vi "Send SMS 2012.vi"(4 "Body":string, 5 "Carrier":enum16{"T-Mobile", "AT&T", "Verizon", "Sprint"}(ring), 6 "Subject":string, 7 "phone number":string, 8 "Error In":errorcluster, 9 "smtp server":string="smtp.gmail.com", 10 "password":string, 11 "email username":string) -> (0 "Error Out":errorcluster)   [LabVIEW 2012]
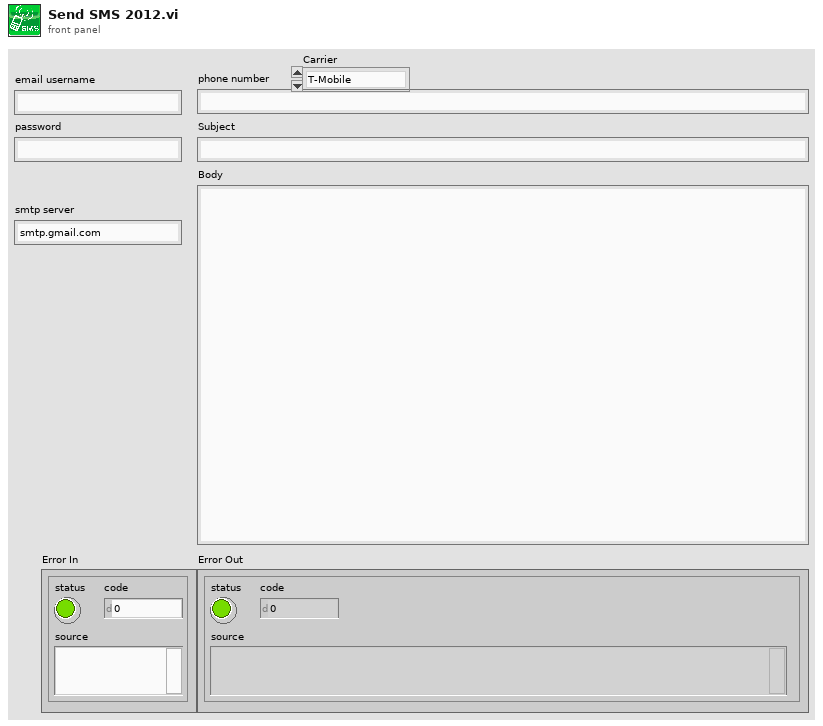
[diagram p1: front panel]
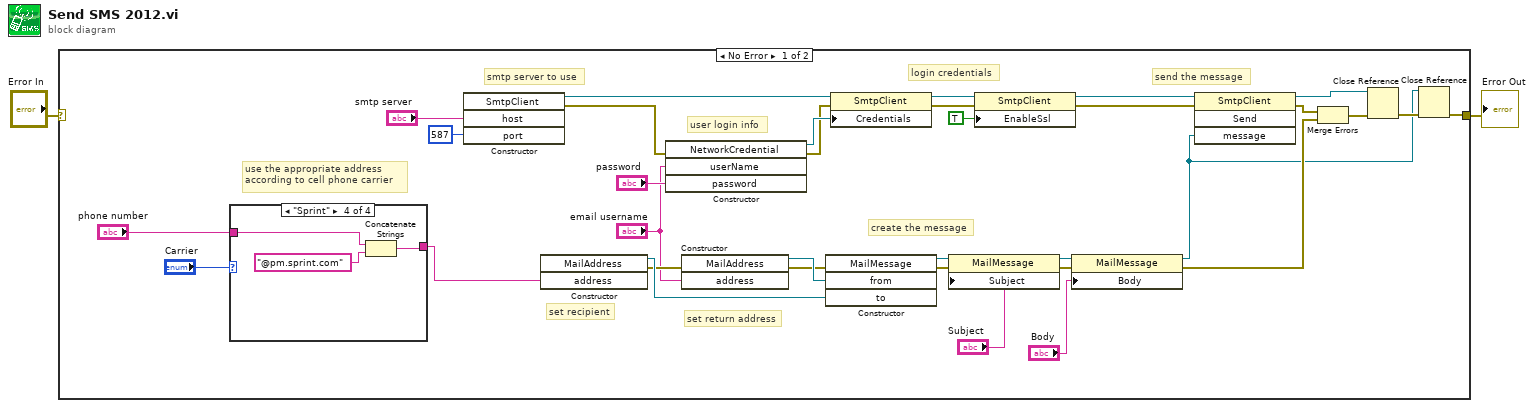
[diagram p0: block diagram]
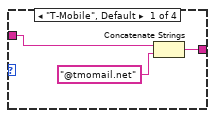
[diagram p2: hidden frame]
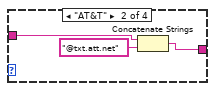
[diagram p3: hidden frame]
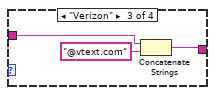
[diagram p4: hidden frame]
diagram:
  n1 = case shown="No Error" "Error In" {
    selector: "Error In" -> [_ w48]
    tunnel: [w4 w48] -> w1
    frame No Error {
      # "user login info"
      # "smtp server to use"
      # "login credentials"
      # "send the message"
      # "create the message"
      # "use the appropriate address\naccording to cell phone carrier"
      # "set return address"
      # "set recipient"
      n2 = case shown="\"Sprint\"" "Carrier" {
        tunnel: "phone number" -> [w38 w40 w43 w46]
        tunnel: [w36 w41 w44 w47] -> w8
        frame "T-Mobile", Default {
          n3 = Concatenate Strings(w38, "@tmomail.net" ("string")) -> (w36:string)
        }
        frame "AT&T" {
          n4 = Concatenate Strings(w40, "@txt.att.net" ("string")) -> (w41:string)
        }
        frame "Verizon" {
          n5 = Concatenate Strings(w43, "@vtext.com" ("string")) -> (w44:string)
        }
        frame "Sprint" {
          n6 = Concatenate Strings(w46, "@pm.sprint.com") -> (w47:string)
        }
      }
      n7 = constructor class="SmtpClient"("host"="smtp server", "port"=587) -> (reference out=w28:refnum<k24>, error out=w21:errorcluster)  [unwired: 3 in, 3 out]
      n8 = constructor class="MailAddress"("address"=w8) -> (reference out=w30:refnum<k24>, error out=w25:errorcluster)  [unwired: 3 in, 2 out]
      n9 = constructor class="NetworkCredential"(error in=w21, "userName"="email username", "password"="password") -> (reference out=w32:refnum<k24>, error out=w20:errorcluster)  [unwired: 2 in, 3 out]
      n10 = constructor class="MailAddress"(error in=w25, "address"="email username") -> (reference out=w31:refnum<k24>, error out=w24:errorcluster)  [unwired: 2 in, 2 out]
      n11 = constructor class="MailMessage"(error in=w24, "from"=w31, "to"=w30) -> (reference out=w29:refnum<k24>, error out=w23:errorcluster)  [unwired: 2 in, 3 out]
      n12 = property class="SmtpClient"(reference=w28, error in=w20, "Credentials"=w32) -> (reference out=w27:refnum<k24>, error out=w19:errorcluster)
      n13 = property class="MailMessage"(reference=w29, error in=w23, "Subject"="Subject") -> (reference out=w35:refnum<k24>, error out=w22:errorcluster)
      n14 = property class="SmtpClient"(reference=w27, error in=w19, "EnableSsl"=TRUE) -> (reference out=w26:refnum<k24>, error out=w18:errorcluster)
      n15 = property class="MailMessage"(reference=w35, error in=w22, "Body"="Body") -> (reference out=w3:refnum<k24>, error out=w17:errorcluster)
      n16 = invoke class="SmtpClient" method="Send"(reference=w26, error in=w18, "message"=w3) -> (reference out=w7:refnum<k24>, error out=w16:errorcluster)  [unwired: 1 in, 2 out]
      n17 = Merge Errors(w16, w17) -> (w6:errorcluster)
      n18 = Close Reference(reference=w7, error in (no error)=w6) -> (error out=w5:errorcluster)
      n19 = Close Reference(reference=w3, error in (no error)=w5) -> (error out=w4:errorcluster)
    }
    frame Error {
    }
  }
  "Error Out" <- w1
